vi "Create (Mode).vi"(8 "error in (no error)":errorcluster, 9 "Mode":string, 10 "Shot":i32, 11 "Name":string) -> (0 "error out":errorcluster, 3 "Tree out":refnum<class "Tree.lvclass">)   [LabVIEW 2012, in "MDSplus.lvlib" / "Tree.lvclass"]
uses:
  <vilib>/MDSplus/Classes/Tree_Class/Tree.lvclass
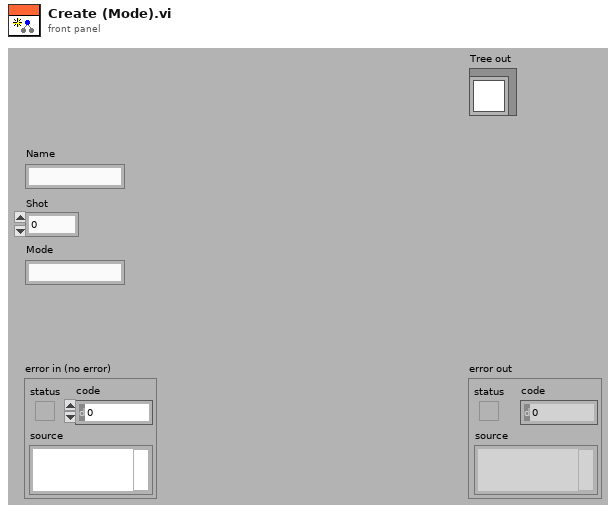
[diagram p1: front panel]
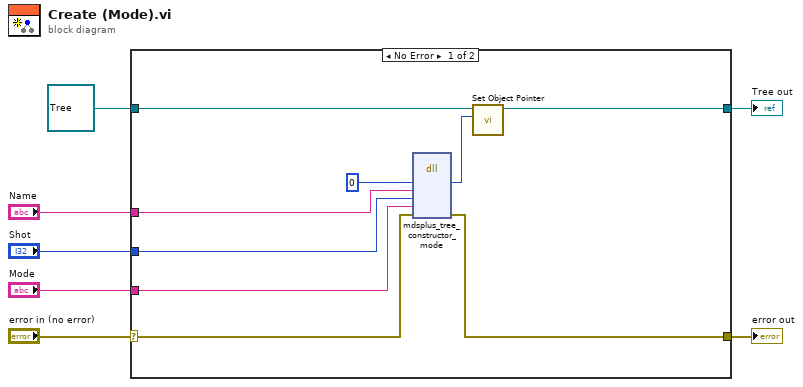
[diagram p0: block diagram]
diagram:
  n1 = case shown="No Error" "error in (no error)" {
    selector: "error in (no error)" -> [w9 w18]
    tunnel: [w8 w18] -> w6
    tunnel: [w11 w17] -> w4
    tunnel: refnum<class "Tree.lvclass"> refnum ("Tree in") -> [w12 w17]
    tunnel: "Name" -> [w15 _]
    tunnel: "Shot" -> [w14 _]
    tunnel: "Mode" -> [w13 _]
    frame No Error {
      n2 = dll-call lib="MDSobjectsLVShr" fn="mdsplus_tree_constructor_mode"("lvTreePtr"=i64 0, "nameIn"=w15, "shotIn"=w14, "modeIn"=w13, "error"=w9) -> ("lvTreePtr"=w10:i64, "error"=w8:errorcluster)  [unwired: 7 in, 2 out]
      n3 = call-dynamic "Set Object Pointer.vi"("Object Pointer"=w10, "Tree in"=w12) -> ("Tree out"=w11:refnum<class "Tree.lvclass">)  [unwired: 9 in]
    }
    frame Error {
    }
  }
  "error out" <- w6
  "Tree out" <- w4
